vi "pixxelAction.vi"(3 "inputArray":u8[](array[numeric]), 4 "u16":u16, 5 "address":string, 6 "playParams":T1, 7 "PIXXELaction":T3=enum."showSceneFrame", 8 "error in (no error)":errorcluster, 9 "location":T2, 10 "color":u32(colorbox), 11 "Pixel-nummer":u8) -> (0 "error out":errorcluster)   [LabVIEW 2014]
uses:
  typeDefs/pixxelAction.ctl
  typeDefs/location.ctl
  typeDefs/playParams.ctl
  typeDefs/poiCommand.ctl
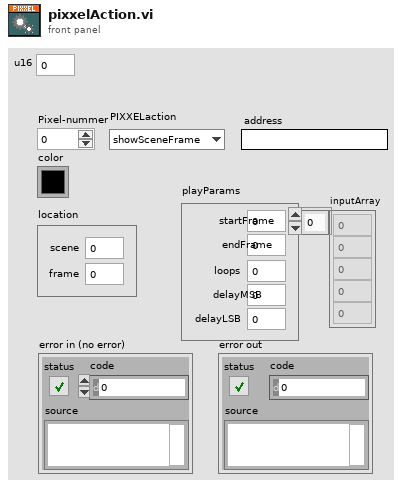
[diagram p1: front panel]
types:
  T1 = typedef "playParams.ctl" = cluster{"startFrame":u8, "endFrame":u8, "loops":u8, "delayMSB":u8, "delayLSB":u8}
  T2 = typedef "location.ctl" = cluster{"scene":u8, "frame":u8}
  T3 = typedef "pixxelAction.ctl" = enum16{"init", "watchdog", "headScene", "setPixel", "tailScene", "headProg", "tailProg", "showSceneFrame", "black", "playFrames", "close", "uploadProg", "startProg", "pauseProg", "stopProg", "jumpTo", "setIP", "setGW", "initFlash", "saveScene", "saveProgram"}
  T4 = typedef "poiCommand.ctl" = u8
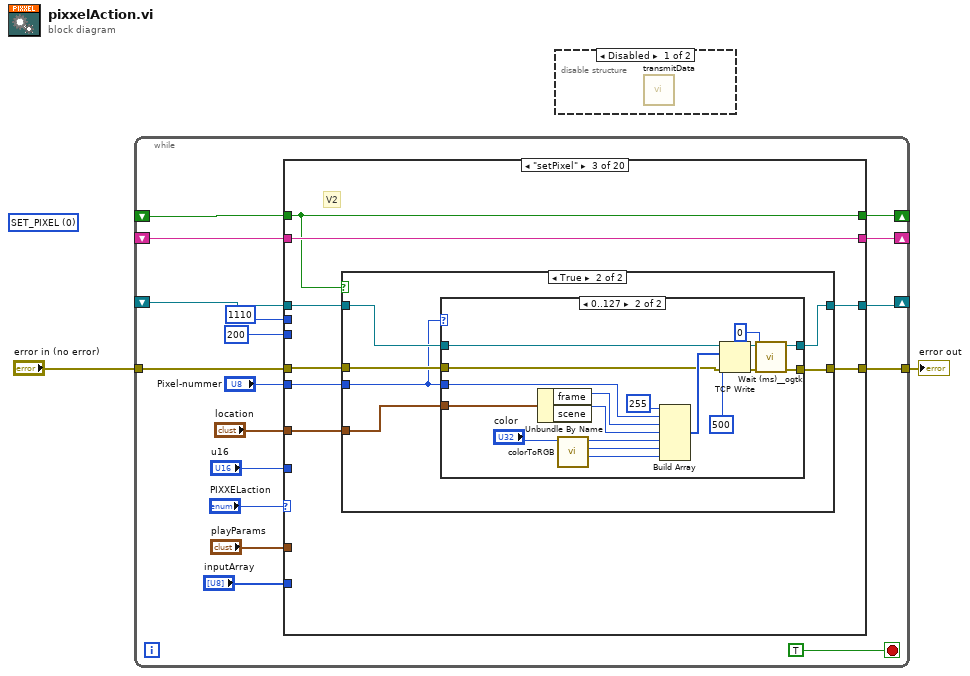
[diagram p0: block diagram]
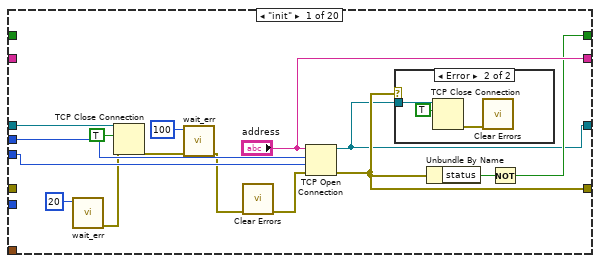
[diagram p3: hidden frame]
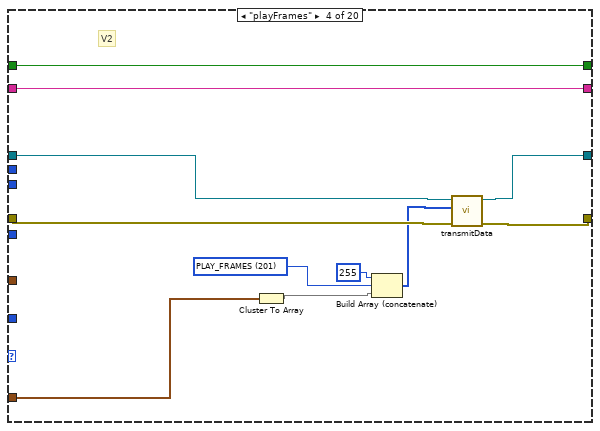
[diagram p8: hidden frame]
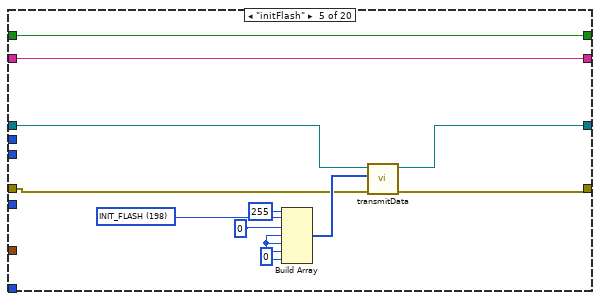
[diagram p9: hidden frame]
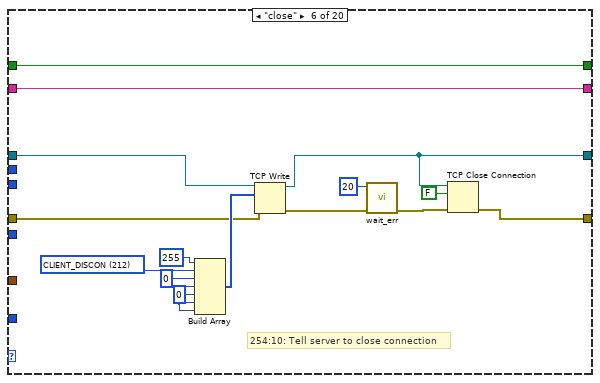
[diagram p10: hidden frame]
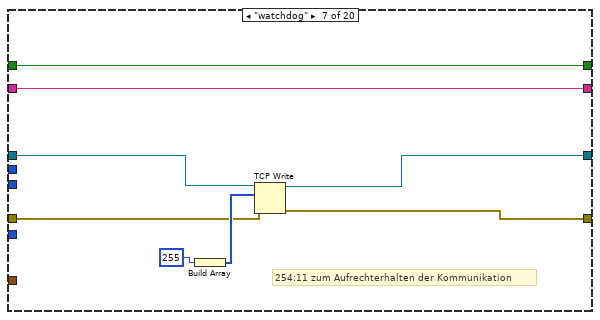
[diagram p11: hidden frame]
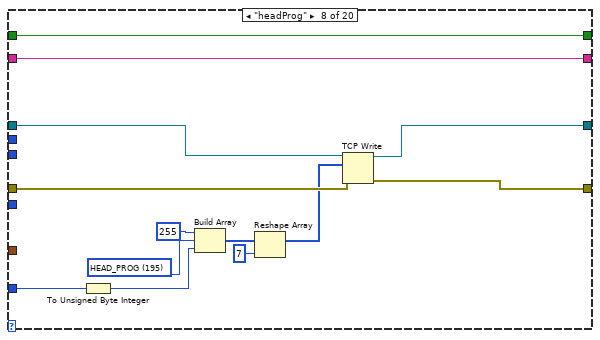
[diagram p12: hidden frame]
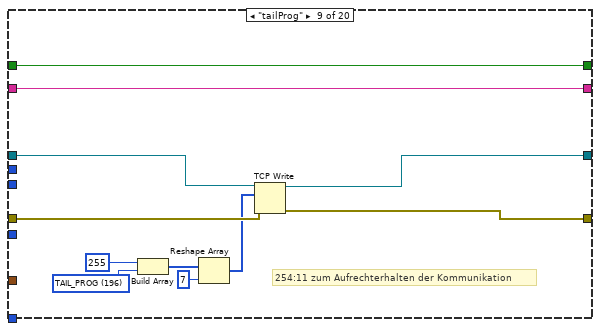
[diagram p13: hidden frame]
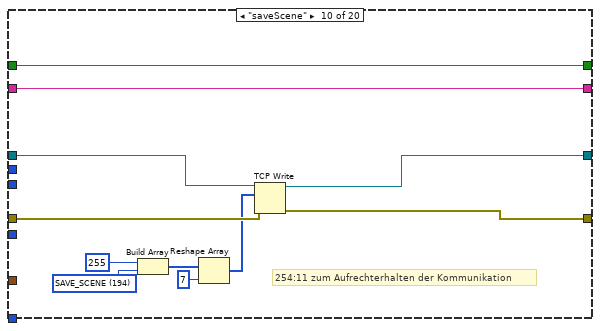
[diagram p14: hidden frame]
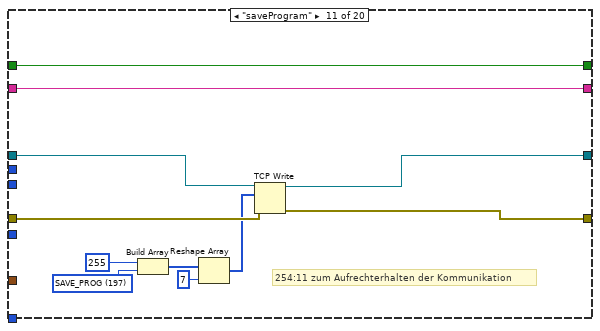
[diagram p15: hidden frame]
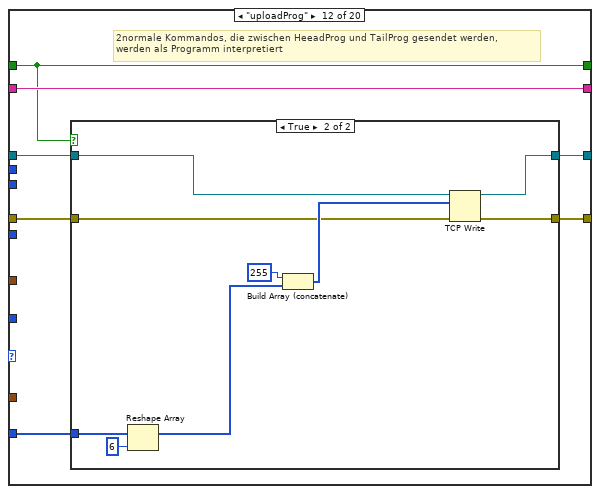
[diagram p16: hidden frame]
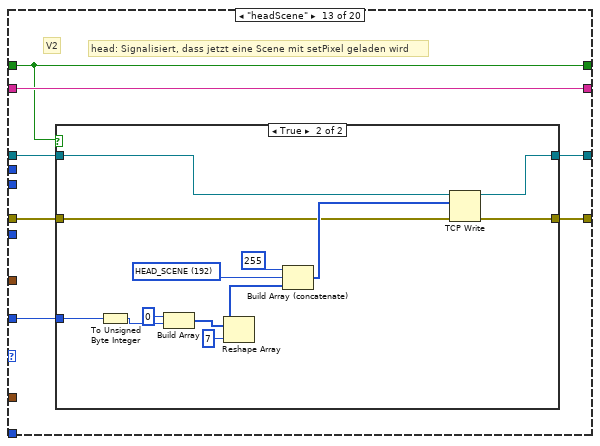
[diagram p18: hidden frame]
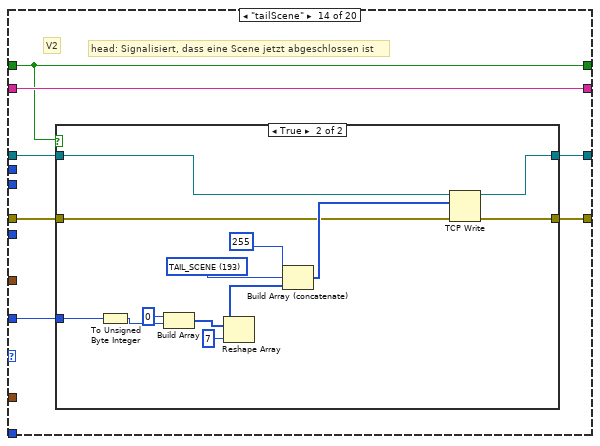
[diagram p20: hidden frame]
diagram:
  (unwired) T4 0 items=["SET_PIXEL"=0, "HEAD_SCENE"=192, "TAIL_SCENE"=193, "SAVE_SCENE"=194, "HEAD_PROG"=195, "TAIL_PROG"=196, "SAVE_PROG"=197, "INIT_FLASH"=198, "LOAD_SCENE"=199, "SHOW_RGB"=200, "PLAY_FRAMES"=201, "ANIMATE"=202, "DISPLAY_IP"=203, "DIMM"=204, "FADE2FRAME"=205, "START_PROG"=206, "STOP_PROC"=207, "PAUSE_PROC"=208, "JUMP2SYNC"=209, "CONNECT"=210, "DISCONNECT"=211, "CLIENT_DISCON"=212, "USE_SSID"=213, "LOOP_START"=214, "SYNC_POINT"=215, "LOOP_END"=216] ("Ring")
  n1 = while {
    shift-right: [w11] -> _
    shift-left: _ -> [w12]
    tunnel: [w16] -> w2
    tunnel: "error in (no error)" -> [w15]
    shift-right: [w8] -> _
    shift-left: _ -> [w7]
    shift-right: [w4] -> _
    shift-left: _ -> [w3]
    stop <- TRUE stop-if-true
    n2 = case shown="\"setPixel\"" "PIXXELaction" {
      tunnel: "Pixel-nummer" -> [_ _ w48 _ _ _ _ _ _ _ _ _ _ _ _ _ _ _ _ _]
      tunnel: [w23 w38 w43 w79 w88 w113 w115 w128 w140 w151 w162 w174 w192 w214 w235 w249 w258 w268 w281 w290] -> w16
      tunnel: w15 -> [_ w38 w47 w78 w89 w106 w118 w131 w143 w154 w165 w173 w191 w213 w234 w248 w257 w267 w280 w289]
      tunnel: "location" -> [_ _ w49 _ _ _ _ _ _ _ _ _ _ _ _ _ _ _ _ _]
      tunnel: "playParams" -> [_ _ _ w86 _ _ _ _ _ _ _ _ _ _ _ _ _ _ _ _]
      tunnel: w12 -> [w34 w41 w46 w81 w91 w104 w117 w130 w142 w153 w164 w172 w190 w212 w233 w251 w260 w270 w279 w288]
      tunnel: [w22 w41 w45 w80 w92 w103 w116 w129 w141 w152 w163 w171 w189 w211 w232 w250 w259 w269 w278 w287] -> w11
      tunnel: u16 1110 ("remote port or service name") -> [w31 _ _ _ _ _ _ _ _ _ _ _ _ _ _ _ _ _ _ _]
      tunnel: 200 ("timeout ms (60000)") -> [w30 _ _ _ _ _ _ _ _ _ _ _ _ _ _ _ _ _ _ _]
      tunnel: ["address" w40 w44 w84 w96 w112 w121 w134 w145 w156 w167 w170 w188 w210 w231 w253 w262 w272 w277 w286] -> w8
      tunnel: w7 -> [_ w40 w44 w84 w96 w112 w121 w134 w145 w156 w167 w170 w188 w210 w231 w253 w262 w272 w277 w286]
      tunnel: "u16" -> [_ _ _ _ _ _ _ w125 _ _ _ _ w187 w209 _ _ _ _ _ _]
      tunnel: "inputArray" -> [_ _ _ _ _ _ _ _ _ _ _ w169 _ _ _ _ _ w263 w274 w283]
      tunnel: [w24 w39 w42 w83 w94 w102 w114 w127 w139 w150 w161 w168 w186 w208 w230 w252 w261 w271 w273 w282] -> w4
      tunnel: w3 -> [_ w39 w42 w83 w94 w102 w114 w127 w139 w150 w161 w168 w186 w208 w230 w252 w261 w271 w273 w282]
      frame "init" {
        n3 = call <userlib>:"wait_err.vi"("milliseconds to wait"=u32 20) -> ("error out"=w21:errorcluster)  [unwired: 10 in]
        n4 = TCP Close Connection(connection ID=w34, abort (F)=TRUE, error in (no error)=w21) -> (error out=w33:errorcluster)  [unwired: 1 out]
        n5 = call <userlib>:"wait_err.vi"("error in (no error)"=w33, "milliseconds to wait"=u32 100) -> ("error out"=w29:errorcluster)  [unwired: 9 in]
        n6 = call <vilib>:"Clear Errors.vi"("error in (no error)"=w29) -> ("error out"=w28:errorcluster)  [unwired: 5 in, 1 out]
        n7 = TCP Open Connection(address="address", remote port or service name=w31, timeout ms (60000)=w30, error in (no error)=w28) -> (connection ID=w22:refnum<k5>, error out=w23:errorcluster)  [unwired: 1 in]
        n8 = case shown="Error" w23 {
          tunnel: w22 -> [_ w37]
          frame No Error {
          }
          frame Error {
            n9 = TCP Close Connection(connection ID=w37, abort (F)=TRUE) -> (error out=w35:errorcluster)  [unwired: 1 in, 1 out]
            n10 = call <vilib>:"Clear Errors.vi"("error in (no error)"=w35) -> ()  [unwired: 5 in, 2 out]
          }
        }
        n11 = Unbundle By Name(w23) -> ("status"=w25:bool)
        n12 = Not(x=w25) -> (.not. x?=w24:bool)
      }
      frame Default {
      }
      frame "setPixel" {
        # "V2"
        n13 = case shown="True" w42 {
          tunnel: w49 -> [_ w57]
          tunnel: w48 -> [_ w52]
          tunnel: w47 -> [w50 w56]
          tunnel: w46 -> [w51 w55]
          tunnel: [w51 w54] -> w45
          tunnel: [w50 w53] -> w43
          frame False {
          }
          frame True {
            n14 = case shown="0..127" w52 {
              tunnel: w57 -> [_ w74]
              tunnel: w52 -> [_ w73]
              tunnel: w56 -> [w58 w69]
              tunnel: w55 -> [w59 w68]
              tunnel: [w59 w67] -> w54
              tunnel: [w58 w66] -> w53
              frame 128, Default {
                # "reserved commands"
              }
              frame 0..127 {
                n15 = Unbundle By Name(w74) -> ("frame"=w72:u8, "scene"=w71:u8)
                n16 = call "colorToRGB.vi"("color"="color") -> ("upper limit"=w60:u8, "upper limit 3"=w61:u8, "upper limit 2"=w62:u8)  [unwired: 8 in]
                n17 = Build Array(u8 255 ("element"), w73, w72, w71, w62, w61, w60) -> (w76:u8[])
                n18 = TCP Write(connection ID=w68, data in=w76, error in (no error)=w69, 9:500 ("timeout ms (25000)")) -> (connection ID out=w67:refnum<k5>, error out=w70:errorcluster)  [unwired: 1 out]
                n19 = call <userlib>:"Wait (ms)__ogtk.vi"("error in (no error)"=w70, "milliseconds to wait"=u32 0) -> ("error out"=w66:errorcluster)  [unwired: 8 in, 1 out]
              }
            }
          }
        }
      }
      frame "playFrames" {
        w82 = T4 201 items=["SET_PIXEL"=0, "HEAD_SCENE"=192, "TAIL_SCENE"=193, "SAVE_SCENE"=194, "HEAD_PROG"=195, "TAIL_PROG"=196, "SAVE_PROG"=197, "INIT_FLASH"=198, "LOAD_SCENE"=199, "SHOW_RGB"=200, "PLAY_FRAMES"=201, "ANIMATE"=202, "DISPLAY_IP"=203, "DIMM"=204, "FADE2FRAME"=205, "START_PROG"=206, "STOP_PROC"=207, "PAUSE_PROC"=208, "JUMP2SYNC"=209, "CONNECT"=210, "DISCONNECT"=211, "CLIENT_DISCON"=212, "USE_SSID"=213, "LOOP_START"=214, "SYNC_POINT"=215, "LOOP_END"=216] ("Ring")
        # "V2"
        n20 = Cluster To Array(cluster=w86) -> (array=w85:u8[])
        n21 = Build Array (concatenate)(u8 255 ("element"), w82, w85) -> (w77:T4[])
        n22 = call "transmitData.vi"("error in (no error)"=w78, "Data"=w77, "TCP Network Connection in"=w81) -> ("error out"=w79:errorcluster, "TCP Network Connection out"=w80:refnum<k5>)  [unwired: 7 in]
      }
      frame "initFlash" {
        w93 = T4 198 items=["SET_PIXEL"=0, "HEAD_SCENE"=192, "TAIL_SCENE"=193, "SAVE_SCENE"=194, "HEAD_PROG"=195, "TAIL_PROG"=196, "SAVE_PROG"=197, "INIT_FLASH"=198, "LOAD_SCENE"=199, "SHOW_RGB"=200, "PLAY_FRAMES"=201, "ANIMATE"=202, "DISPLAY_IP"=203, "DIMM"=204, "FADE2FRAME"=205, "START_PROG"=206, "STOP_PROC"=207, "PAUSE_PROC"=208, "JUMP2SYNC"=209, "CONNECT"=210, "DISCONNECT"=211, "CLIENT_DISCON"=212, "USE_SSID"=213, "LOOP_START"=214, "SYNC_POINT"=215, "LOOP_END"=216] ("Ring")
        w95 = u8 0 ("element")
        n23 = Build Array(u8 255 ("element"), w93, u8 0 ("element"), w95, w95, w95, w95) -> (w90:T4[])
        n24 = call "transmitData.vi"("error in (no error)"=w89, "Data"=w90, "TCP Network Connection in"=w91) -> ("error out"=w88:errorcluster, "TCP Network Connection out"=w92:refnum<k5>)  [unwired: 7 in]
      }
      frame "close" {
        w99 = T4 212 items=["SET_PIXEL"=0, "HEAD_SCENE"=192, "TAIL_SCENE"=193, "SAVE_SCENE"=194, "HEAD_PROG"=195, "TAIL_PROG"=196, "SAVE_PROG"=197, "INIT_FLASH"=198, "LOAD_SCENE"=199, "SHOW_RGB"=200, "PLAY_FRAMES"=201, "ANIMATE"=202, "DISPLAY_IP"=203, "DIMM"=204, "FADE2FRAME"=205, "START_PROG"=206, "STOP_PROC"=207, "PAUSE_PROC"=208, "JUMP2SYNC"=209, "CONNECT"=210, "DISCONNECT"=211, "CLIENT_DISCON"=212, "USE_SSID"=213, "LOOP_START"=214, "SYNC_POINT"=215, "LOOP_END"=216] ("Ring")
        w108 = u8 0 ("element")
        # "254:10: Tell server to close connection"
        n25 = Build Array(u8 255 ("element"), w99, u8 0 ("element"), w108, w108, w108, w108) -> (w109:T4[])
        n26 = TCP Write(connection ID=w104, data in=w109, error in (no error)=w106) -> (connection ID out=w103:refnum<k5>, error out=w105:errorcluster)  [unwired: 1 in, 1 out]
        n27 = call <userlib>:"wait_err.vi"("error in (no error)"=w105, "milliseconds to wait"=u32 20) -> ("error out"=w101:errorcluster)  [unwired: 9 in]
        n28 = TCP Close Connection(connection ID=w103, abort (F)=FALSE, error in (no error)=w101) -> (error out=w113:errorcluster)  [unwired: 1 out]
      }
      frame "watchdog" {
        # "254:11 zum Aufrechterhalten der Kommunikation"
        n29 = Build Array(u8 255 ("element")) -> (w119:u8[])
        n30 = TCP Write(connection ID=w117, data in=w119, error in (no error)=w118) -> (connection ID out=w116:refnum<k5>, error out=w115:errorcluster)  [unwired: 1 in, 1 out]
      }
      frame "headProg" {
        w126 = T4 195 items=["SET_PIXEL"=0, "HEAD_SCENE"=192, "TAIL_SCENE"=193, "SAVE_SCENE"=194, "HEAD_PROG"=195, "TAIL_PROG"=196, "SAVE_PROG"=197, "INIT_FLASH"=198, "LOAD_SCENE"=199, "SHOW_RGB"=200, "PLAY_FRAMES"=201, "ANIMATE"=202, "DISPLAY_IP"=203, "DIMM"=204, "FADE2FRAME"=205, "START_PROG"=206, "STOP_PROC"=207, "PAUSE_PROC"=208, "JUMP2SYNC"=209, "CONNECT"=210, "DISCONNECT"=211, "CLIENT_DISCON"=212, "USE_SSID"=213, "LOOP_START"=214, "SYNC_POINT"=215, "LOOP_END"=216] ("Ring")
        n31 = To Unsigned Byte Integer(number=w125) -> (unsigned 8bit integer=w124:u8)
        n32 = Build Array(u8 255 ("element"), w126, w124) -> (w132:T4[])
        n33 = Reshape Array(w132, 7 ("dimension size")) -> (w123:T4[])
        n34 = TCP Write(connection ID=w130, data in=w123, error in (no error)=w131) -> (connection ID out=w129:refnum<k5>, error out=w128:errorcluster)  [unwired: 1 in, 1 out]
      }
      frame "tailProg" {
        w138 = T4 196 items=["SET_PIXEL"=0, "HEAD_SCENE"=192, "TAIL_SCENE"=193, "SAVE_SCENE"=194, "HEAD_PROG"=195, "TAIL_PROG"=196, "SAVE_PROG"=197, "INIT_FLASH"=198, "LOAD_SCENE"=199, "SHOW_RGB"=200, "PLAY_FRAMES"=201, "ANIMATE"=202, "DISPLAY_IP"=203, "DIMM"=204, "FADE2FRAME"=205, "START_PROG"=206, "STOP_PROC"=207, "PAUSE_PROC"=208, "JUMP2SYNC"=209, "CONNECT"=210, "DISCONNECT"=211, "CLIENT_DISCON"=212, "USE_SSID"=213, "LOOP_START"=214, "SYNC_POINT"=215, "LOOP_END"=216] ("Ring")
        # "254:11 zum Aufrechterhalten der Kommunikation"
        n35 = Build Array(u8 255 ("element"), w138) -> (w137:T4[])
        n36 = Reshape Array(w137, 7 ("dimension size")) -> (w136:T4[])
        n37 = TCP Write(connection ID=w142, data in=w136, error in (no error)=w143) -> (connection ID out=w141:refnum<k5>, error out=w140:errorcluster)  [unwired: 1 in, 1 out]
      }
      frame "saveScene" {
        w149 = T4 194 items=["SET_PIXEL"=0, "HEAD_SCENE"=192, "TAIL_SCENE"=193, "SAVE_SCENE"=194, "HEAD_PROG"=195, "TAIL_PROG"=196, "SAVE_PROG"=197, "INIT_FLASH"=198, "LOAD_SCENE"=199, "SHOW_RGB"=200, "PLAY_FRAMES"=201, "ANIMATE"=202, "DISPLAY_IP"=203, "DIMM"=204, "FADE2FRAME"=205, "START_PROG"=206, "STOP_PROC"=207, "PAUSE_PROC"=208, "JUMP2SYNC"=209, "CONNECT"=210, "DISCONNECT"=211, "CLIENT_DISCON"=212, "USE_SSID"=213, "LOOP_START"=214, "SYNC_POINT"=215, "LOOP_END"=216] ("Ring")
        # "254:11 zum Aufrechterhalten der Kommunikation"
        n38 = Build Array(u8 255 ("element"), w149) -> (w148:T4[])
        n39 = Reshape Array(w148, 7 ("dimension size")) -> (w147:T4[])
        n40 = TCP Write(connection ID=w153, data in=w147, error in (no error)=w154) -> (connection ID out=w152:refnum<k5>, error out=w151:errorcluster)  [unwired: 1 in, 1 out]
      }
      frame "saveProgram" {
        w160 = T4 197 items=["SET_PIXEL"=0, "HEAD_SCENE"=192, "TAIL_SCENE"=193, "SAVE_SCENE"=194, "HEAD_PROG"=195, "TAIL_PROG"=196, "SAVE_PROG"=197, "INIT_FLASH"=198, "LOAD_SCENE"=199, "SHOW_RGB"=200, "PLAY_FRAMES"=201, "ANIMATE"=202, "DISPLAY_IP"=203, "DIMM"=204, "FADE2FRAME"=205, "START_PROG"=206, "STOP_PROC"=207, "PAUSE_PROC"=208, "JUMP2SYNC"=209, "CONNECT"=210, "DISCONNECT"=211, "CLIENT_DISCON"=212, "USE_SSID"=213, "LOOP_START"=214, "SYNC_POINT"=215, "LOOP_END"=216] ("Ring")
        # "254:11 zum Aufrechterhalten der Kommunikation"
        n41 = Build Array(u8 255 ("element"), w160) -> (w159:T4[])
        n42 = Reshape Array(w159, 7 ("dimension size")) -> (w158:T4[])
        n43 = TCP Write(connection ID=w164, data in=w158, error in (no error)=w165) -> (connection ID out=w163:refnum<k5>, error out=w162:errorcluster)  [unwired: 1 in, 1 out]
      }
      frame "uploadProg" {
        # "2normale Kommandos, die zwischen HeeadProg und TailProg gesendet werden,\nwerden als Programm interpretiert"
        n44 = case shown="True" w168 {
          tunnel: [w175 w183] -> w174
          tunnel: w173 -> [w175 w182]
          tunnel: w172 -> [w176 w181]
          tunnel: [w176 w180] -> w171
          tunnel: w169 -> [_ w179]
          frame False {
          }
          frame True {
            n45 = Reshape Array(w179, 6 ("dimension size")) -> (w178:u8[])
            n46 = Build Array (concatenate)(u8 255 ("element"), w178) -> (w184:u8[])
            n47 = TCP Write(connection ID=w181, data in=w184, error in (no error)=w182) -> (connection ID out=w180:refnum<k5>, error out=w183:errorcluster)  [unwired: 1 in, 1 out]
          }
        }
      }
      frame "headScene" {
        # "V2"
        # "head: Signalisiert, dass jetzt eine Scene mit setPixel geladen wird"
        n48 = case shown="True" w186 {
          tunnel: [w193 w206] -> w192
          tunnel: w191 -> [w193 w205]
          tunnel: w190 -> [w194 w204]
          tunnel: [w194 w203] -> w189
          tunnel: w187 -> [_ w198]
          frame False {
          }
          frame True {
            w196 = T4 192 items=["SET_PIXEL"=0, "HEAD_SCENE"=192, "TAIL_SCENE"=193, "SAVE_SCENE"=194, "HEAD_PROG"=195, "TAIL_PROG"=196, "SAVE_PROG"=197, "INIT_FLASH"=198, "LOAD_SCENE"=199, "SHOW_RGB"=200, "PLAY_FRAMES"=201, "ANIMATE"=202, "DISPLAY_IP"=203, "DIMM"=204, "FADE2FRAME"=205, "START_PROG"=206, "STOP_PROC"=207, "PAUSE_PROC"=208, "JUMP2SYNC"=209, "CONNECT"=210, "DISCONNECT"=211, "CLIENT_DISCON"=212, "USE_SSID"=213, "LOOP_START"=214, "SYNC_POINT"=215, "LOOP_END"=216] ("Ring")
            n49 = To Unsigned Byte Integer(number=w198) -> (unsigned 8bit integer=w197:u8)
            n50 = Build Array(u8 0 ("element"), w197) -> (w200:u8[])
            n51 = Reshape Array(w200, 7 ("dimension size")) -> (w202:u8[])
            n52 = Build Array (concatenate)(u8 255 ("element"), w196, w202) -> (w207:T4[])
            n53 = TCP Write(connection ID=w204, data in=w207, error in (no error)=w205) -> (connection ID out=w203:refnum<k5>, error out=w206:errorcluster)  [unwired: 1 in, 1 out]
          }
        }
      }
      frame "tailScene" {
        # "V2"
        # "head: Signalisiert, dass eine Scene jetzt abgeschlossen ist"
        n54 = case shown="True" w208 {
          tunnel: [w215 w228] -> w214
          tunnel: w213 -> [w215 w227]
          tunnel: w212 -> [w216 w226]
          tunnel: [w216 w225] -> w211
          tunnel: w209 -> [_ w220]
          frame False {
          }
          frame True {
            w218 = T4 193 items=["SET_PIXEL"=0, "HEAD_SCENE"=192, "TAIL_SCENE"=193, "SAVE_SCENE"=194, "HEAD_PROG"=195, "TAIL_PROG"=196, "SAVE_PROG"=197, "INIT_FLASH"=198, "LOAD_SCENE"=199, "SHOW_RGB"=200, "PLAY_FRAMES"=201, "ANIMATE"=202, "DISPLAY_IP"=203, "DIMM"=204, "FADE2FRAME"=205, "START_PROG"=206, "STOP_PROC"=207, "PAUSE_PROC"=208, "JUMP2SYNC"=209, "CONNECT"=210, "DISCONNECT"=211, "CLIENT_DISCON"=212, "USE_SSID"=213, "LOOP_START"=214, "SYNC_POINT"=215, "LOOP_END"=216] ("Ring")
            n55 = To Unsigned Byte Integer(number=w220) -> (unsigned 8bit integer=w219:u8)
            n56 = Build Array(u8 0 ("element"), w219) -> (w222:u8[])
            n57 = Reshape Array(w222, 7 ("dimension size")) -> (w224:u8[])
            n58 = Build Array (concatenate)(u8 255 ("element"), w218, w224) -> (w229:T4[])
            n59 = TCP Write(connection ID=w226, data in=w229, error in (no error)=w227) -> (connection ID out=w225:refnum<k5>, error out=w228:errorcluster)  [unwired: 1 in, 1 out]
          }
        }
      }
      frame "startProg" {
        # "V2"
        n60 = case shown="True" w230 {
          tunnel: [w236 w244] -> w235
          tunnel: w234 -> [w236 w243]
          tunnel: w233 -> [w237 w242]
          tunnel: [w237 w241] -> w232
          frame False {
          }
          frame True {
            w240 = T4 206 items=["SET_PIXEL"=0, "HEAD_SCENE"=192, "TAIL_SCENE"=193, "SAVE_SCENE"=194, "HEAD_PROG"=195, "TAIL_PROG"=196, "SAVE_PROG"=197, "INIT_FLASH"=198, "LOAD_SCENE"=199, "SHOW_RGB"=200, "PLAY_FRAMES"=201, "ANIMATE"=202, "DISPLAY_IP"=203, "DIMM"=204, "FADE2FRAME"=205, "START_PROG"=206, "STOP_PROC"=207, "PAUSE_PROC"=208, "JUMP2SYNC"=209, "CONNECT"=210, "DISCONNECT"=211, "CLIENT_DISCON"=212, "USE_SSID"=213, "LOOP_START"=214, "SYNC_POINT"=215, "LOOP_END"=216] ("Ring")
            n61 = Build Array(u8 255, w240) -> (w238:T4[])
            n62 = call "transmitData.vi"("error in (no error)"=w243, "Data"=w238, "TCP Network Connection in"=w242) -> ("error out"=w244:errorcluster, "TCP Network Connection out"=w241:refnum<k5>)  [unwired: 7 in]
          }
        }
      }
      frame "pauseProg" {
        w246 = T4 208 items=["SET_PIXEL"=0, "HEAD_SCENE"=192, "TAIL_SCENE"=193, "SAVE_SCENE"=194, "HEAD_PROG"=195, "TAIL_PROG"=196, "SAVE_PROG"=197, "INIT_FLASH"=198, "LOAD_SCENE"=199, "SHOW_RGB"=200, "PLAY_FRAMES"=201, "ANIMATE"=202, "DISPLAY_IP"=203, "DIMM"=204, "FADE2FRAME"=205, "START_PROG"=206, "STOP_PROC"=207, "PAUSE_PROC"=208, "JUMP2SYNC"=209, "CONNECT"=210, "DISCONNECT"=211, "CLIENT_DISCON"=212, "USE_SSID"=213, "LOOP_START"=214, "SYNC_POINT"=215, "LOOP_END"=216] ("Ring")
        # "V2"
        n63 = Build Array(u8 255 ("element"), w246) -> (w245:T4[])
        n64 = call "transmitData.vi"("error in (no error)"=w248, "Data"=w245, "TCP Network Connection in"=w251) -> ("error out"=w249:errorcluster, "TCP Network Connection out"=w250:refnum<k5>)  [unwired: 7 in]
      }
      frame "stopProg" {
        w255 = T4 207 items=["SET_PIXEL"=0, "HEAD_SCENE"=192, "TAIL_SCENE"=193, "SAVE_SCENE"=194, "HEAD_PROG"=195, "TAIL_PROG"=196, "SAVE_PROG"=197, "INIT_FLASH"=198, "LOAD_SCENE"=199, "SHOW_RGB"=200, "PLAY_FRAMES"=201, "ANIMATE"=202, "DISPLAY_IP"=203, "DIMM"=204, "FADE2FRAME"=205, "START_PROG"=206, "STOP_PROC"=207, "PAUSE_PROC"=208, "JUMP2SYNC"=209, "CONNECT"=210, "DISCONNECT"=211, "CLIENT_DISCON"=212, "USE_SSID"=213, "LOOP_START"=214, "SYNC_POINT"=215, "LOOP_END"=216] ("Ring")
        # "V2"
        n65 = Build Array(u8 255 ("element"), w255) -> (w254:T4[])
        n66 = call "transmitData.vi"("error in (no error)"=w257, "Data"=w254, "TCP Network Connection in"=w260) -> ("error out"=w258:errorcluster, "TCP Network Connection out"=w259:refnum<k5>)  [unwired: 7 in]
      }
      frame "jumpTo" {
        w265 = T4 209 items=["SET_PIXEL"=0, "HEAD_SCENE"=192, "TAIL_SCENE"=193, "SAVE_SCENE"=194, "HEAD_PROG"=195, "TAIL_PROG"=196, "SAVE_PROG"=197, "INIT_FLASH"=198, "LOAD_SCENE"=199, "SHOW_RGB"=200, "PLAY_FRAMES"=201, "ANIMATE"=202, "DISPLAY_IP"=203, "DIMM"=204, "FADE2FRAME"=205, "START_PROG"=206, "STOP_PROC"=207, "PAUSE_PROC"=208, "JUMP2SYNC"=209, "CONNECT"=210, "DISCONNECT"=211, "CLIENT_DISCON"=212, "USE_SSID"=213, "LOOP_START"=214, "SYNC_POINT"=215, "LOOP_END"=216] ("Ring")
        # "V2"
        n67 = Build Array (concatenate)(u8 255 ("element"), w265, w263) -> (w264:T4[])
        n68 = call "transmitData.vi"("error in (no error)"=w267, "Data"=w264, "TCP Network Connection in"=w270) -> ("error out"=w268:errorcluster, "TCP Network Connection out"=w269:refnum<k5>)  [unwired: 7 in]
      }
      frame "setIP" {
        n69 = Build Array (concatenate)(u8[] [255, 254, 7], w274) -> (w275:u8[])
        n70 = TCP Write(connection ID=w279, data in=w275, error in (no error)=w280) -> (connection ID out=w278:refnum<k5>, error out=w281:errorcluster)  [unwired: 1 in, 1 out]
      }
      frame "setGW" {
        n71 = Build Array (concatenate)(u8[] [255, 254, 8], w283) -> (w284:u8[])
        n72 = TCP Write(connection ID=w288, data in=w284, error in (no error)=w289) -> (connection ID out=w287:refnum<k5>, error out=w290:errorcluster)  [unwired: 1 in, 1 out]
      }
    }
  }
  "error out" <- w2
  n73 = disable-structure shown="Disabled" {
    frame Disabled {
      n74 = call "transmitData.vi"() -> ()  [unwired: 10 in, 2 out]
    }
    frame Enabled {
    }
  }
